vi "Handle setConfiguration.vi"(8 "error in (no error)":errorcluster, 10 "setConfiguration":variant, 11 "Inst.Magneto in":refnum<class "Inst.Magneto.lvclass">) -> (0 "error out":errorcluster, 3 "Inst.Magneto out":refnum<class "Inst.Magneto.lvclass">)   [LabVIEW 2019, in "Inst.Magneto.lvclass"]
uses:
  Inst.Magneto.lvclass
  Inst.Magneto.lvclass/Inst.Magneto.ctl
  45e4b271-6884-462c-ad3a-d505ab08eb62.vi
  45e4b271-6884-462c-ad3a-d505ab08eb62.vi/1bcccaf9-4497-409c-b794-abe9adbe854f.vi
  45e4b271-6884-462c-ad3a-d505ab08eb62.vi/7fb63b73-6614-449d-8556-fd5cf15ed521.vi
  <vilib>/Utility/Data Type/Get Type Information.vi
  <vilib>/JDP Science/JSONtext/JSON text to Variant.vi
  <vilib>/JDP Science/JSONtext/LVClass Serializer/JSONtext LVClass Serializer.lvclass
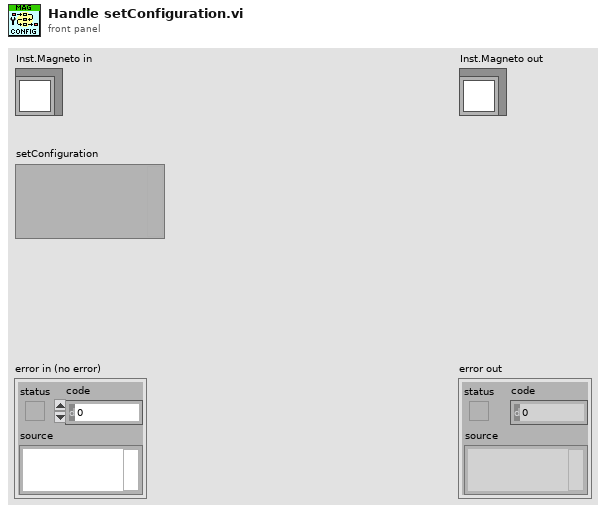
[diagram p1: front panel]
types:
  T1 = typedef "Inst.Magneto.lvclass/Inst.Magneto.Configuration--Cluster.ctl" = cluster{"Server URL":string}
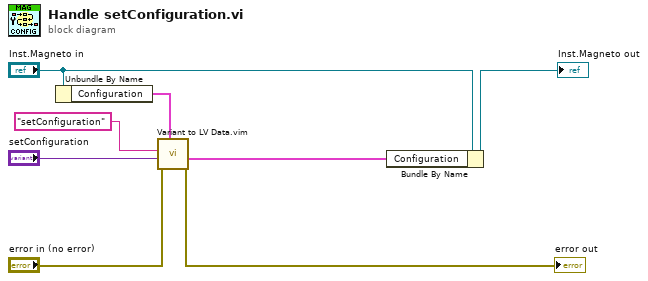
[diagram p0: block diagram]
diagram:
  n1 = Unbundle By Name("Inst.Magneto in") -> ("Configuration"=w7:T1)
  n2 = call "Variant to LV Data.vim"("type"=w7, "error in (no error)"="error in (no error)", "JSON Data in"="setConfiguration", "Command"="setConfiguration") -> ("error out"=→"error out":errorcluster, "Data out"=w1:T1)  [unwired: 4 in, 2 out]
  n3 = Bundle By Name(cluster="Inst.Magneto in", "Configuration"=w1) -> (→"Inst.Magneto out":refnum<class "Inst.Magneto.lvclass">)
